vi "Launch.vi"(8 "error in (no error)":errorcluster, 10 "User Interface":refnum<class "User Interface.lvclass">, 11 "User Interface Handler in":refnum<class "User Interface Handler.lvclass">) -> (0 "error out":errorcluster, 2 "active vi":T1, 3 "User Interface Handler out":refnum<class "User Interface Handler.lvclass">)   [LabVIEW 2017, in "DSF Core.lvlib" / "User Interface Handler.lvclass"]
uses:
  User Interface Handler.lvclass
  User Interface/User Interface.lvclass
  User Interface Ref.ctl
  User Interface Handler.lvclass/User Interface Handler.ctl
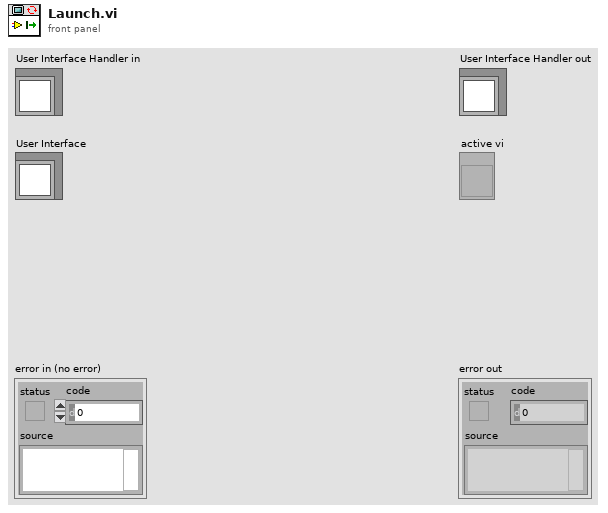
[diagram p1: front panel]
types:
  T1 = typedef "DSF Core.lvlib/User Interface Handler.lvclass/User Interface Ref.ctl" = refnum<vi>
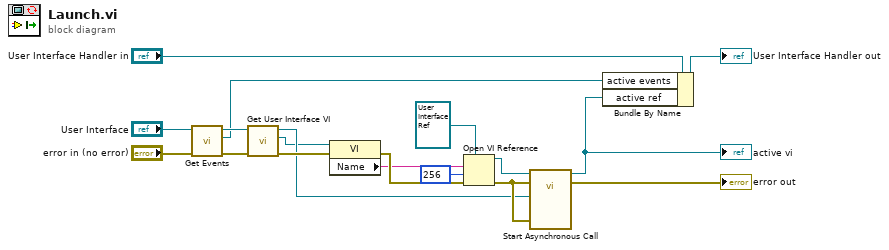
[diagram p0: block diagram]
diagram:
  n1 = call "Get Events.vi"("error in (no error)"="error in (no error)", "User Interface in"="User Interface") -> ("error out"=w7:errorcluster, "events"=w4:refnum<class "User Interface Events.lvclass">, "User Interface out"=w5:refnum<class "User Interface.lvclass">)  [unwired: 7 in]
  n2 = call-dynamic "Get User Interface VI.vi"("error in (no error)"=w7, "User Interface in"=w5) -> ("error out"=w12:errorcluster, "user interface vi"=w9:refnum<vi>, "User Interface out"=w11:refnum<class "User Interface.lvclass">)  [unwired: 7 in]
  n3 = property class="VI"(reference=w9, error in=w12) -> (error out=w15:errorcluster, "Name"=w14:string)  [unwired: 1 out]
  n4 = Open VI Reference(type specifier VI Refnum (for type only)=T1 refnum, vi path=w14, options=256, error in (no error)=w15) -> (vi reference=w13:T1, error out=w17:errorcluster)  [unwired: 2 in]
  n5 = call-by-ref "Start Asynchronous Call"(reference=w13, error in=w17, 8:"error in (no error)"=w17, "User Interface in"=w11) -> (reference out=w3:T1, error out=→"error out":errorcluster)  [unwired: 8 in, 2 out]
  "active vi" <- w3
  n6 = Bundle By Name(cluster="User Interface Handler in", "active events"=w4, "active ref"=w3) -> (→"User Interface Handler out":refnum<class "User Interface Handler.lvclass">)
